vi "Initialize.vi"(8 "error in (no error)":errorcluster, 10 "Stage Comms":T1={"CommsProtocol.lvclass"=refnum, "CommsProtocol.lvclass 2"=refnum, "CommsProtocol.lvclass 3"=refnum, "XYZ Control Config"=enum."XYZ", "Translation Stage Description"=""}, 11 "Scientifica XYZ Gen1 in":refnum<class "Scientifica XYZ Gen1.lvclass">) -> (0 "error out":errorcluster, 3 "Scientifica XYZ Gen1 out":refnum<class "Scientifica XYZ Gen1.lvclass">)   [LabVIEW 2020, in "TranslationStageClassStructure.lvlib" / "Scientifica XYZ Gen1.lvclass"]
uses:
  Scientifica XYZ Gen1.lvclass
  typedefs/TranslationStageControlInfo.ctl
  Generic Comms/CommsProtocol/CommsProtocol.lvclass
  typedefs/XYZControlConfig.ctl
  Serial Comms/Serial Comms/Serial Comms.lvclass
  Scientifica XYZ Gen1.lvclass/Scientifica XYZ Gen1.ctl
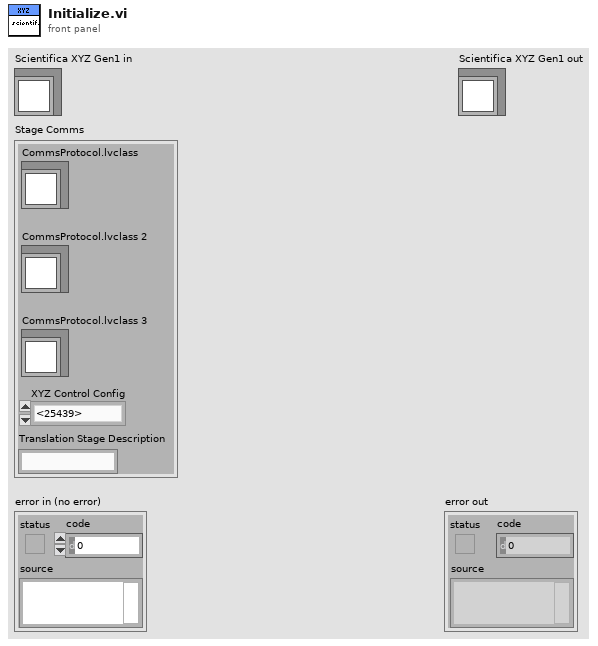
[diagram p1: front panel]
types:
  T1 = typedef "TranslationStageControlInfo.ctl" = cluster{"CommsProtocol.lvclass":refnum<class "CommsProtocol.lvclass">, "CommsProtocol.lvclass 2":refnum<class "CommsProtocol.lvclass">, "CommsProtocol.lvclass 3":refnum<class "CommsProtocol.lvclass">, "XYZ Control Config":T2, "Translation Stage Description":string}
  T2 = typedef "XYZControlConfig.ctl" = enum16{"None", "XYZ", "XY-Z", "X-Y-Z", "Z"}
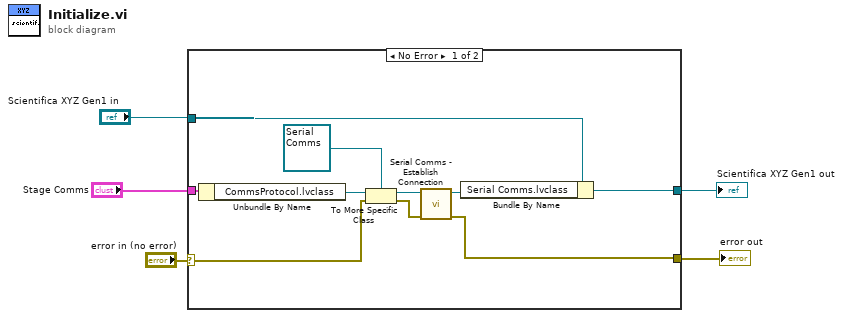
[diagram p0: block diagram]
diagram:
  n1 = case shown="No Error" "error in (no error)" {
    selector: "error in (no error)" -> [w8 w17]
    tunnel: [w12 w17] -> w4
    tunnel: [w14 w16] -> w2
    tunnel: "Scientifica XYZ Gen1 in" -> [w15 w16]
    tunnel: "Stage Comms" -> [w11 _]
    frame No Error {
      n2 = Unbundle By Name(w11) -> ("CommsProtocol.lvclass"=w10:refnum<class "CommsProtocol.lvclass">)
      n3 = To More Specific Class(target class=refnum<class "Serial Comms.lvclass"> refnum ("Serial Comms.lvclass"), reference=w10, error in=w8) -> (specific class reference=w6:refnum<class "Serial Comms.lvclass">, error out=w7:errorcluster)
      n4 = call "Serial Comms - Establish Connection.vi"("error in (no error)"=w7, "Serial Comms in"=w6) -> ("error out"=w12:errorcluster, "Serial Comms out"=w13:refnum<class "Serial Comms.lvclass">)  [unwired: 8 in]
      n5 = Bundle By Name(cluster=w15, "Serial Comms.lvclass"=w13) -> (w14:refnum<class "Scientifica XYZ Gen1.lvclass">)
    }
    frame Error {
    }
  }
  "error out" <- w4
  "Scientifica XYZ Gen1 out" <- w2
